vi "Script - copy frame.vi"(5 "FrameNames":string[](array[string]), 7 "Array":i32[](array[numeric]), 8 "error in":errorcluster, 9 "Structure Type":T1, 10 "Numeric":i32, 11 "StructRef":refnum<vi>) -> (0 "error out":errorcluster)   [LabVIEW 2020]
uses:
  StructureTypes.ctl
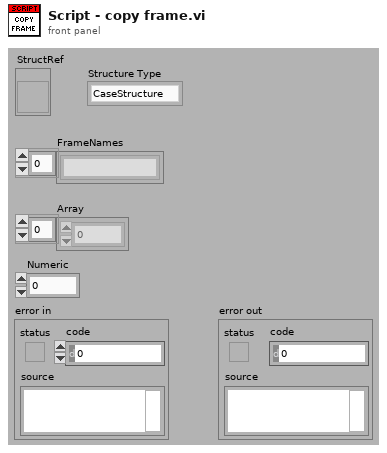
[diagram p1: front panel]
types:
  T1 = typedef "StructureTypes.ctl" = enum16{"CaseStructure", "EventStructure"}
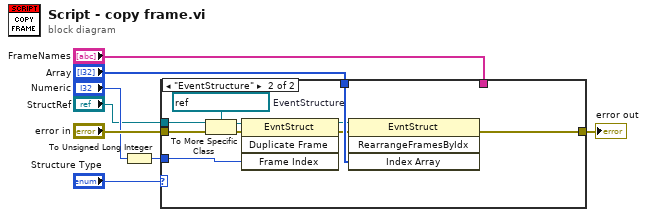
[diagram p0: block diagram]
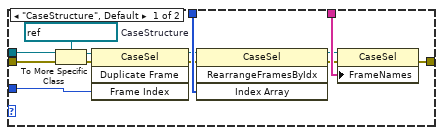
[diagram p2: hidden frame]
diagram:
  n1 = To Unsigned Long Integer(number="Numeric") -> (unsigned 32bit integer=w2:u32)
  n2 = case shown="\"EventStructure\"" "Structure Type" {
    tunnel: "FrameNames" -> [w21 _]
    tunnel: [w20 w22] -> w7
    tunnel: "Array" -> [w17 w31]
    tunnel: "error in" -> [w12 w26]
    tunnel: "StructRef" -> [w9 w23]
    tunnel: w2 -> [w16 w30]
    frame "CaseStructure", Default {
      w13 = refnum<vi> refnum  # CaseStructure
      n3 = To More Specific Class(target class=w13, reference=w9, error in=w12) -> (specific class reference=w10:refnum<vi>, error out=w11:errorcluster)
      n4 = invoke class="CaseSel" method="Duplicate Frame"(reference=w10, error in=w11, "Frame Index"=w16) -> (reference out=w15:refnum<vi>, error out=w14:errorcluster)  [unwired: 1 in, 2 out]
      n5 = invoke class="CaseSel" method="RearrangeFramesByIdx"(reference=w15, error in=w14, "Index Array"=w17) -> (reference out=w19:refnum<vi>, error out=w18:errorcluster)  [unwired: 1 in, 2 out]
      n6 = property class="CaseSel"(reference=w19, error in=w18, "FrameNames"=w21) -> (error out=w20:errorcluster)  [unwired: 1 out]
    }
    frame "EventStructure" {
      w27 = refnum<vi> refnum  # EventStructure
      n7 = To More Specific Class(target class=w27, reference=w23, error in=w26) -> (specific class reference=w24:refnum<vi>, error out=w25:errorcluster)
      n8 = invoke class="EvntStruct" method="Duplicate Frame"(reference=w24, error in=w25, "Frame Index"=w30) -> (reference out=w29:refnum<vi>, error out=w28:errorcluster)  [unwired: 1 in, 2 out]
      n9 = invoke class="EvntStruct" method="RearrangeFramesByIdx"(reference=w29, error in=w28, "Index Array"=w31) -> (error out=w22:errorcluster)  [unwired: 1 in, 3 out]
    }
  }
  "error out" <- w7
